vi "Calculate Accel Distances.vi"(9 "Length (f)":dbl, 10 "Velocities":dbl[](array[numeric]), 11 "Limits":T2) -> (3 "Distances":T1(array[cluster]), 5 "Const V Dist":T1(array[cluster]))   [LabVIEW 2019]
uses:
  Globals.vi
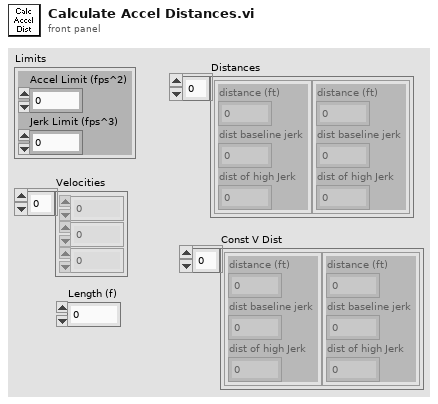
[diagram p1: front panel]
types:
  T1 = cluster{"distance (ft)":dbl, "dist baseline jerk":dbl, "dist of high Jerk":dbl}[]
  T2 = cluster{"Accel Limit (fps^2)":dbl, "Jerk Limit (fps^3)":dbl}
  T3 = cluster{"distance (ft)":dbl, "dist baseline jerk":dbl, "dist of high Jerk":dbl}
  T4 = cluster{"distance (ft)":i32, "dist baseline jerk":i32, "dist of high Jerk":i32}
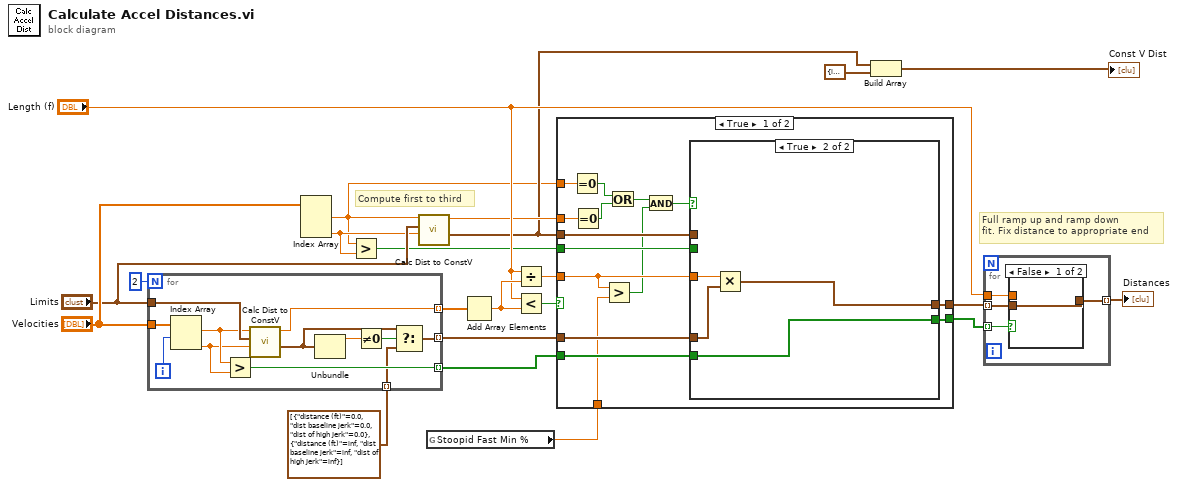
[diagram p0: block diagram]
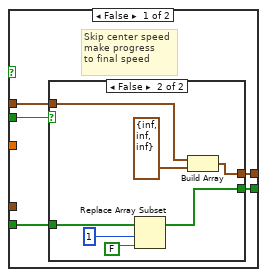
[diagram p2: hidden frame]
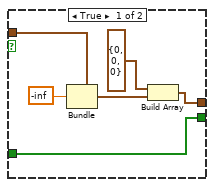
[diagram p3: hidden frame]
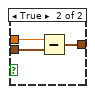
[diagram p5: hidden frame]
diagram:
  # "Compute first to third"
  # "Full ramp up and ramp down\nfit. Fix distance to appropriate end"
  n1 = for {
    N: 2 -> [_]
    tunnel: "Velocities" -> [w34]
    tunnel: "Limits" -> [w33]
    tunnel: [w30] -> w18 mode=indexing
    tunnel: [w25] -> w10 mode=indexing
    tunnel: T1 [{"distance (ft)"=0.0, "dist baseline jerk"=0.0, "dist of high Jerk"=0.0}, {"distance (ft)"=inf, "dist baseline jerk"=inf, "dist of high Jerk"=inf}] -> [w24] mode=indexing
    tunnel: [w23] -> w13 mode=indexing
    i -> [w27]
    n2 = Index Array(array=w34, index #1=w27) -> (element #1=w32:dbl, element #2=w31:dbl)  [unwired: 1 in]
    n3 = Greater?(x=w32, y=w31) -> (0:w25:bool)
    n4 = call "Calc Dist to ConstV.vi"("V2 (fps)"=w31, "Limits"=w33, "V1  (fps)"=w32) -> ("distances"=w29:T3, "distance (ft)"=w23:dbl)  [unwired: 6 in, 1 out]
    n5 = Unbundle(w29) -> ("distance (ft)"=w26:dbl)  [unwired: 2 out]
    n6 = Not Equal To 0?(x=w26) -> (x != 0?=w28:bool)
    n7 = Select(t=w29, s=w28, f=w24) -> (s? t:f=w30:T3)
  }
  n8 = Index Array(array="Velocities") -> (element #1=w2:dbl, element #3=w4:dbl)  [unwired: 3 in, 1 out]
  n9 = Greater?(x=w2, y=w4) -> (0:w3:bool)
  n10 = call "Calc Dist to ConstV.vi"("V2 (fps)"=w4, "Limits"="Limits", "V1  (fps)"=w2) -> ("distances"=w5:T3, "distance (ft)"=w8:dbl)  [unwired: 6 in, 1 out]
  n11 = global read "Globals.vi" "Stoopid Fast Min %"() -> (w1:dbl)
  n12 = Add Array Elements(numeric array=w13) -> (sum=w12:dbl)
  n13 = Divide(x="Length (f)", y=w12) -> (x/y=w19:dbl)
  n14 = Less?(x="Length (f)", y=w12) -> (x < y?=w16:bool)
  n15 = case shown="True" w16 {
    tunnel: w19 -> [w39 _]
    tunnel: w18 -> [w43 w73]
    tunnel: [w49 w73] -> w17
    tunnel: w10 -> [w47 w72]
    tunnel: [w46 w72] -> w9
    tunnel: w5 -> [w48 _]
    tunnel: w8 -> [w44 _]
    tunnel: w3 -> [w45 _]
    tunnel: w2 -> [w40 _]
    tunnel: w1 -> [w38 _]
    frame True {
      n16 = Equal To 0?(x=w40) -> (x = 0?=w42:bool)
      n17 = Equal To 0?(x=w44) -> (x = 0?=w41:bool)
      n18 = Greater?(x=w39, y=w38) -> (0:w37:bool)
      n19 = Or(x=w42, y=w41) -> (x .or. y?=w36:bool)
      n20 = And(x=w36, y=w37) -> (x .and. y?=w35:bool)
      n21 = case shown="True" w35 {
        tunnel: [w54 w69] -> w49
        tunnel: w48 -> [w53 _]
        tunnel: w47 -> [w52 w68]
        tunnel: [w51 w68] -> w46
        tunnel: w45 -> [w50 _]
        tunnel: w43 -> [_ w70]
        tunnel: w39 -> [_ w71]
        frame False {
          # "Skip center speed\nmake progress\nto final speed"
          n22 = case shown="False" w50 {
            tunnel: [w60 w67] -> w54
            tunnel: w53 -> [w57 w66]
            tunnel: w52 -> [w55 w65]
            tunnel: [w55 w63] -> w51
            frame True {
              n23 = Bundle(cluster=w57, "dist baseline jerk"=-inf) -> (w58:T3)  [unwired: 2 in]
              n24 = Build Array(T4 {"distance (ft)"=0, "dist baseline jerk"=0, "dist of high Jerk"=0} ("distances"), w58) -> (w60:T1)
            }
            frame False {
              n25 = Replace Array Subset(array=w65, new element=FALSE, index=1) -> (w63:bool[])
              n26 = Build Array(w66, T3 {"distance (ft)"=inf, "dist baseline jerk"=inf, "dist of high Jerk"=inf} ("distances")) -> (w67:T1)
            }
          }
        }
        frame True {
          n27 = Multiply(x=w71, y=w70) -> (x*y=w69:T1)
        }
      }
    }
    frame False {
      # "Trapezoid or full triangle"
    }
  }
  n28 = Build Array(w5, T3 {"distance (ft)"=inf, "dist baseline jerk"=inf, "dist of high Jerk"=inf} ("distances")) -> (→"Const V Dist":T1)
  n29 = for {
    tunnel: w9 -> [w77] mode=indexing
    tunnel: w17 -> [w75] mode=indexing
    tunnel: "Length (f)" -> [w76]
    tunnel: [w74] -> w21 mode=indexing
    n30 = case shown="False" w77 {
      tunnel: w76 -> [_ w81]
      tunnel: w75 -> [w78 w80]
      tunnel: [w78 w79] -> w74
      frame False {
      }
      frame True {
        n31 = Subtract(x=w81, y=w80) -> (x-y=w79:T3)
      }
    }
  }
  "Distances" <- w21
